vi "Periodic Trigger__ogtk.vi"(7 "time (ms)":u32, 9 "reset":bool) -> (6 "Triggered":bool, 8 "time since last call":u32, 10 "timer value":u32)   [LabVIEW 2014]
doc: "This VI will periodically output a Boolean TRUE on a specified time interval. The internal timer's counter can be reset to zero, via the \"reset\" Boolean input."
panel:
  # "[OpenG VI Tags] ***Do Not Remove***"
  # "Periodic Trigger.vi\n\nThis VI will periodically output a Boolean TRUE on a specified time interval.\n\nPlease visit http://www.OpenG.org to learn about the\nOpen Source LabVIEW software movement.\n\nNOTICE -- YOU MUST LEAVE THIS NOTICE IN PLACE.  PER THE TERMS OF THE LICENSE BELOW, YOU MAY SUBLICENSE THIS SOFTWARE \nIN ANY WAY THAT DOES NOT CONFLICT WITH THIS LICENSE.\n\n### BSD License (http://www.opensource.org/licenses/bsd-license.php) Begin ###\n \nCopyright (c) 2002, Jim Kring <jim@jimkring.com>\n\nAll rights reserved.\n\nRedistribution and use in source and binary forms, with or without modification, are permitted provided that the following conditions are met:\n\n    * Redistributions of source code must retain the above copyright notice, this list of conditions and the following disclaimer.\n    * Redistributions in binary form must reproduce the above copyright notice, this list of conditions and the following disclaimer in the \n       documentation and/or other materials provided with the distribution.\n    * Neither the name of SciWare, James Kring, Inc., nor the names of its contributors may be used to endorse or promote products derived \n       from this software without specific prior written permission.\n\nTHIS SOFTWARE IS PROVIDED BY THE COPYRIGHT HOLDERS AND CONTRIBUTORS \"AS IS\" AND ANY EXPRESS OR IMPLIED WARRANTIES, \nINCLUDING, BUT NOT LIMITED TO, THE IMPLIED WARRANTIES OF MERCHANTABILITY AND FITNESS FOR A PARTICULAR PURPOSE ARE \nDISCLAIMED. IN NO EVENT SHALL THE COPYRIGHT OWNER OR CONTRIBUTORS BE LIABLE FOR ANY DIRECT, INDIRECT, INCIDENTAL,\n SPECIAL, EXEMPLARY, OR CONSEQUENTIAL DAMAGES (INCLUDING, BUT NOT LIMITED TO, PROCUREMENT OF SUBSTITUTE GOODS OR \nSERVICES; LOSS OF USE, DATA, OR PROFITS; OR BUSINESS INTERRUPTION) HOWEVER CAUSED AND ON ANY THEORY OF LIABILITY, \nWHETHER IN CONTRACT, STRICT LIABILITY, OR TORT (INCLUDING NEGLIGENCE OR OTHERWISE) ARISING IN ANY WAY OUT OF THE USE \nOF THIS SOFTWARE, EVEN IF ADVISED OF THE POSSIBILITY OF SUCH DAMAGE.\n\n### BSD License End ###"
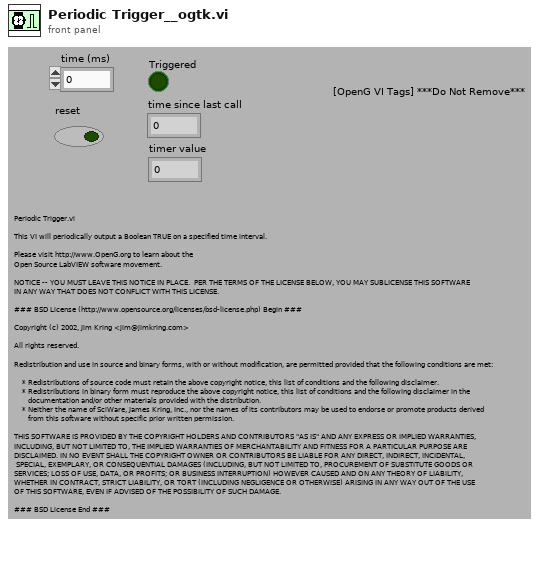
[diagram p1: front panel]
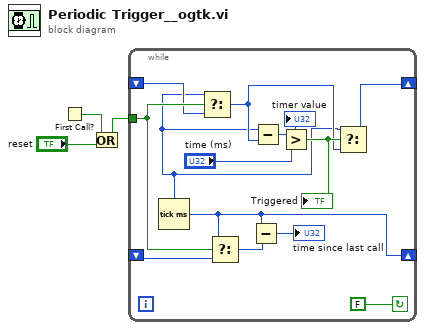
[diagram p0: block diagram]
diagram:
  n1 = First Call?() -> (First Call?: T/F=w3:bool)
  n2 = Or(x=w3, y="reset") -> (x .or. y?=w1:bool)
  n3 = while {
    shift-left: _ -> [w10]
    shift-right: [w4] -> _
    shift-left: _ -> [w7]
    shift-right: [w12] -> _
    tunnel: w1 -> [w8]
    stop <- FALSE continue-if-true
    n4 = Tick Count (ms)() -> (millisecond timer value=w4:u32)
    n5 = Select(t=w4, s=w8, f=w7) -> (s? t:f=w6:u32)
    n6 = Select(t=w4, s=w8, f=w10) -> (s? t:f=w5:u32)
    n7 = Subtract(x=w4, y=w5) -> (x-y=→"time since last call":u32)
    n8 = Subtract(x=w4, y=w6) -> (x-y=w15:u32)
    "timer value" <- w15
    n9 = Greater?(x=w15, y="time (ms)") -> (0:w13:bool)
    "Triggered" <- w13
    n10 = Select(t=w4, s=w13, f=w6) -> (s? t:f=w12:u32)
  }
